vi "给行上色.vi"(6 "列数":i32, 8 "错误输入（无错误）":errorcluster, 9 "选中颜色盒":u32(colorbox)=12439011, 10 "坐标":T1={"Row"=20, "Column"=20} caption="本次坐标", 11 "引用输入":refnum<vi>) -> (0 "错误输出":errorcluster, 3 "引用输出":refnum<vi>)   [LabVIEW 2014, in "表格.lvlib" / "表格上色.lvlib"]
uses:
  <vilib>/Utility/miscctls.llb/LVRowAndColumnTypeDef.ctl
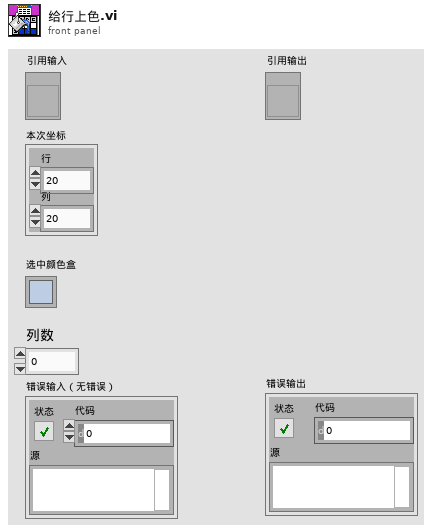
[diagram p1: front panel]
types:
  T1 = typedef "LVRowAndColumnTypeDef.ctl" = cluster{"Row":i32, "Column":i32}
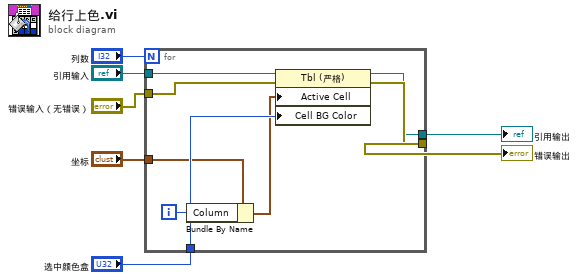
[diagram p0: block diagram]
diagram:
  n1 = for {
    N: "列数" -> [_]
    tunnel: "选中颜色盒" -> [w15]
    tunnel: [w14] -> w7
    tunnel: "坐标" -> [w12]
    tunnel: [w13] -> w5
    tunnel: "引用输入" -> [w9]
    tunnel: "错误输入（无错误）" -> [w8]
    i -> [w11]
    n2 = Bundle By Name(cluster=w12, "Column"=w11) -> (w10:T1)
    n3 = property on="属性节点" class="Tbl (严格)"(reference=w9, error in=w8, "Active Cell"=w10, "Cell BG Color"=w15) -> (reference out=w13:refnum<vi>, error out=w14:errorcluster)
  }
  "错误输出" <- w7
  "引用输出" <- w5
